vi "lvEtherbone.device_close.vi"(0 "eb_socket_ID":i32, 1 "eb_device_ID":i32, 5 "error in (no error)":errorcluster) -> (13 "eb_status":T1, 14 "eb_socket_ID out":i32, 19 "error out":errorcluster)   [LabVIEW 2009, in "lvEtherbone.lvlib"]
doc: "//-----------------------------------------------------------------------------------\n// author : Dietrich Beck, GSI-Darmstadt\n// purpose : Close a remote Etherbone device.\n// returns : lveb_status_t\n//-----------------------------------------------------------------------------------\nETHERBONE_API int lveb_device_close(int eb_deviceID //ID of Wishbone devie\n );"
uses:
  lvEtherbone.lvlib
  lvEtherbone.lveb_status_t.ctl
  bin/lvEtherbone.dll
panel:
  in  "eb_status_t":T1
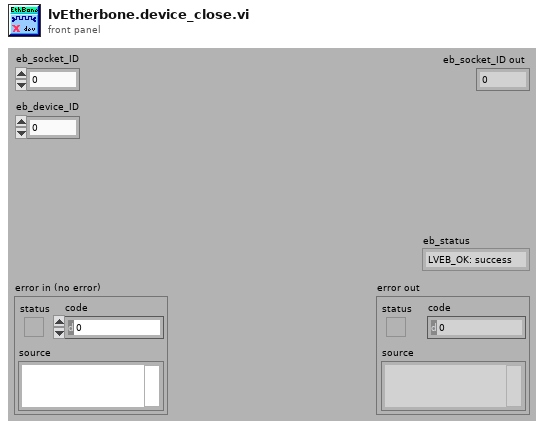
[diagram p1: front panel]
types:
  T1 = typedef "lvEtherbone.lvlib/lvEtherbone.lveb_status_t.ctl" = enum32{"LVEB_OK: success", "LVEB_UNKNOWN: unknown error", "LVEB_OS: operating system forbids access", "LVEB_PORT: port in use or unavailable", "LVEB_ID: ID invalid or out of resources", "LVEB_SOCKET: socket invalid or unavailable", "LVEB_EB: remote address is not Etherbone conformant", "LVEB_IP: bad format or network address", "LVEB_BUSWIDTH: bus width error", "LVEB_DEVICEBUSY: Whishbone device still busy", "LVEB_DEVICEFAIL: operation on Wishbone device failed", "LVEB_DEVICEEXIST: Whishbone device already exists, overlaps, or does not exist", "LVEB_TIMEDOUT: a timeout occurred", "LVEB_OVERFLOW: payload of Etherbone exceeded", "LVEB_ADDRESS: bad address"}
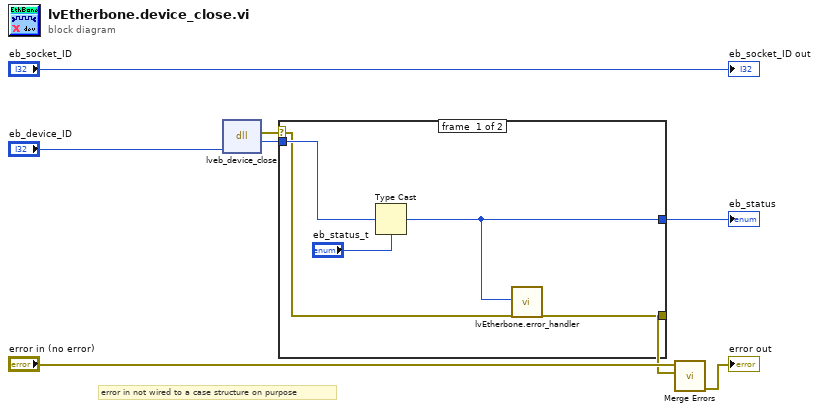
[diagram p0: block diagram]
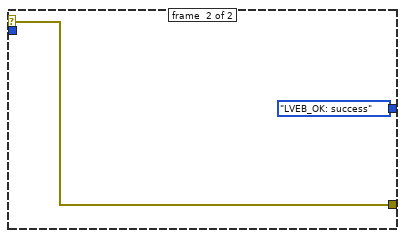
[diagram p2: hidden frame]
diagram:
  # "error in not wired to a case structure on purpose"
  n1 = dll-call lib="F:/beck/Project/BEL/SCC/etherbone-core/api/lvEtherbone/bin/lvEtherbone.*" fn="lveb_device_close"("eb_device_ID"="eb_device_ID") -> (error out=w5:errorcluster, "eb_status"=w6:i32)  [unwired: 4 in, 1 out]
  n2 = case shown="No Error" w5 {
    selector: w5 -> [w9 w15]
    tunnel: w6 -> [w13 _]
    tunnel: [w11 lvEtherbone.lveb_status_t."LVEB_OK: success" ("eb_status_t")] -> w8
    tunnel: [w10 w15] -> w3
    frame #0 {
      n3 = Type Cast(type="eb_status_t", x=w13) -> (*(type *) &x=w11:T1)
      n4 = call "lvEtherbone.error_handler.vi"("eb_status"=w11, "error in"=w9) -> ("error out"=w10:errorcluster)  [unwired: 17 in]
    }
    frame #1 {
    }
  }
  "eb_status" <- w8
  n5 = call <vilib>:"Merge Errors.vi"("error in 2 (no error)"=w3, "error in 1 (no error)"="error in (no error)") -> ("error out"=→"error out":errorcluster)  [unwired: 5 in]
  "eb_socket_ID out" <- "eb_socket_ID"
